vi "S30c_dll F73.vi"(4 "error in":errorcluster, 6 "Channel":enum16{"CH0", "P1", "P2", "T", "TOB1", "TOB2"}(ring), 7 "Dev Addr":u8=250) -> (0 "error out":errorcluster, 2 "Status":u8 format="%.0b", 3 "Value":sgl)   [LabVIEW 2014, in "K_S30c_dll.lvlib"]
uses:
  K_S30c_dll.lvlib
  s30c.dll
panel:
  # "Function 73: read value\n\nusing s30c.dll\nKeller AG für Druckmesstechnik, 29.5.08 b.v."
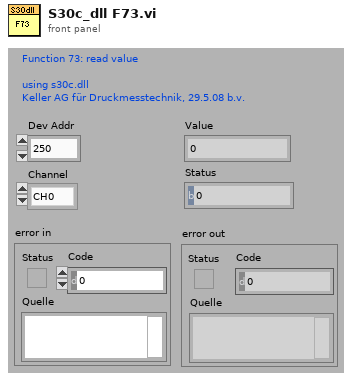
[diagram p1: front panel]
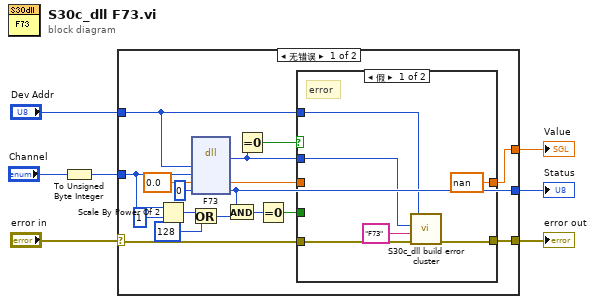
[diagram p0: block diagram]
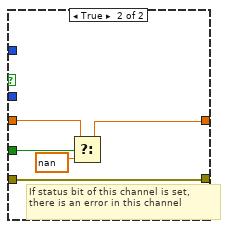
[diagram p2: hidden frame]
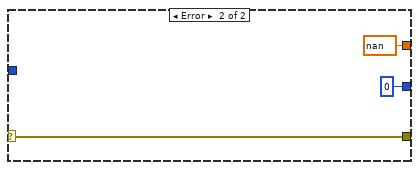
[diagram p3: hidden frame]
diagram:
  n1 = To Unsigned Byte Integer(number="Channel") -> (unsigned 8bit integer=w1:u8)
  n2 = case shown="无错误" "error in" {
    selector: "error in" -> [w19 w38]
    tunnel: [w22 w38] -> w7
    tunnel: "Dev Addr" -> [w16 _]
    tunnel: w1 -> [w14 _]
    tunnel: [w17 sgl nan ("Value")] -> w5
    tunnel: [w11 u8 0 ("Status")] -> w4
    frame No Error {
      n3 = Scale By Power Of 2(n=w14, x=u8 1) -> (x*2^n=w10:u8)
      n4 = Or(x=w10, y=u8 128) -> (x .or. y?=w9:u8)
      n5 = dll-call lib="PTH2Labs EworkSINOPEC北控自动相渗software2.08.5_dlls30c.dll" fn="F73" label="dll call F73"("DevAddr"=w16, "Channel"=w14, "Value"=sgl 0.0, "Status"=u8 0) -> ("Rückgabetyp"=w21:i16, "Value"=w18:sgl, "Status"=w11:u8)  [unwired: 5 in, 2 out]
      n6 = And(x=w11, y=w9) -> (x .and. y?=w13:u8)
      n7 = Equal To 0?(x=w21) -> (x = 0?=w24:bool)
      n8 = Equal To 0?(x=w13) -> (x = 0?=w12:bool)
      n9 = case shown="假" w24 {
        tunnel: w19 -> [w29 w31]
        tunnel: [w28 w31] -> w22
        tunnel: w21 -> [w27 _]
        tunnel: w18 -> [_ w34]
        tunnel: [sgl nan ("Value") w33] -> w17
        tunnel: w16 -> [w25 _]
        tunnel: w12 -> [_ w35]
        frame False {
          # "error"
          n10 = call "S30c_dll build error cluster.vi"("error in"=w29, "error Text"="F73", "error code"=w27, "Dev Addr"=w25) -> ("error out"=w28:errorcluster)  [unwired: 3 in]
        }
        frame True {
          # "If status bit of this channel is set,\nthere is an error in this channel"
          n11 = Select(t=w34, s=w35, f=sgl nan ("Value")) -> (s? t:f=w33:sgl)
        }
      }
    }
    frame Error {
    }
  }
  "error out" <- w7
  "Value" <- w5
  "Status" <- w4
